vi "Test Read SD and MCP4725.vi"() -> ()   [LabVIEW 2014]
uses:
  <vilib>/LabVIEW Universal Transcriptor/MCP4725/MCP4725.lvclass
  <vilib>/LabVIEW Universal Transcriptor/LabVIEW to Arduino Transcriptor/Transcriptors/System API/Serial println string.vi
  <vilib>/LabVIEW Universal Transcriptor/LabVIEW to Arduino Transcriptor/Transcriptors/System API/Serial print integer.vi
  <vilib>/LabVIEW Universal Transcriptor/LabVIEW to Arduino Transcriptor/Transcriptors/System API/Serial print string.vi
  <vilib>/LabVIEW Universal Transcriptor/LabVIEW Universal Transcriptor SD Card Library/File.lvclass
  <vilib>/LabVIEW Universal Transcriptor/LabVIEW Universal Transcriptor SD Card Library/LabVIEW Universal Transcriptor SD Card Library.lvlib
  <vilib>/LabVIEW Universal Transcriptor/LabVIEW to Arduino Transcriptor/Transcriptors/System API/System Serial Library Variables/System Serial Library Variables.lvlib
panel:
  out "success?":bool
  out "String Buffer":string
  in  "Error In":errorcluster
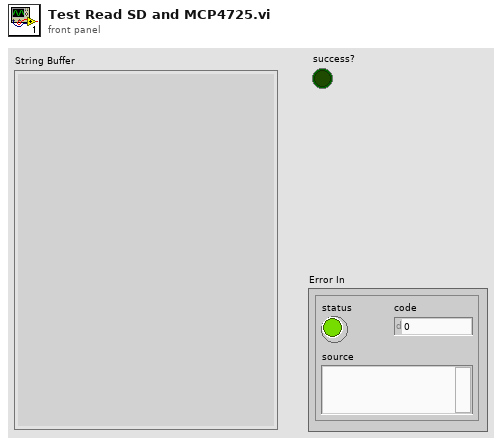
[diagram p1: front panel]
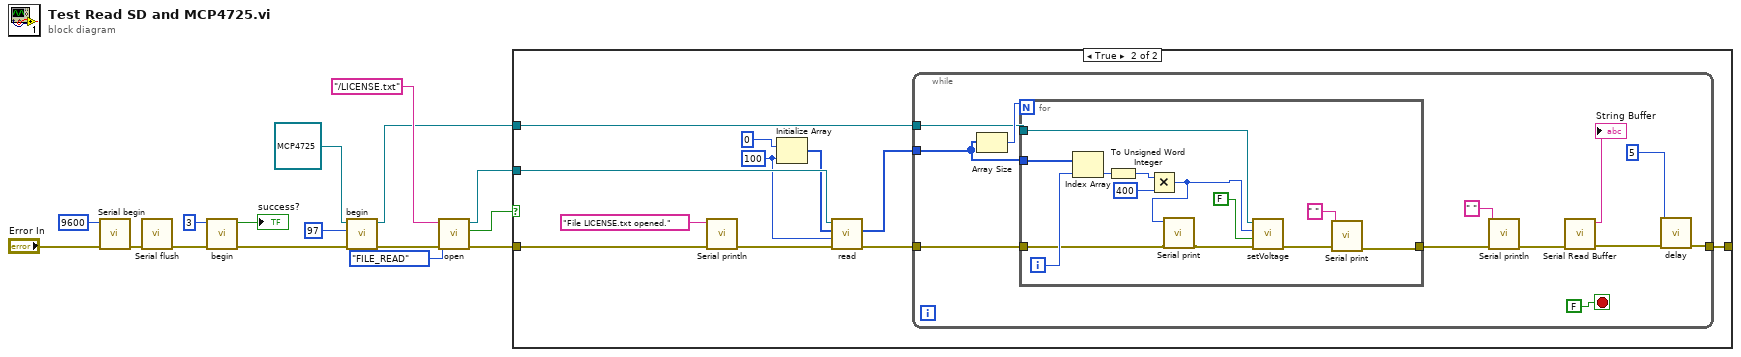
[diagram p0: block diagram]
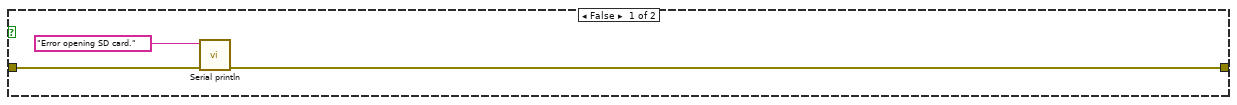
[diagram p2: hidden frame]
diagram:
  n1 = call <vilib>:"Serial begin.vi"("Error In"="Error In", "speed (Bd)"=9600) -> ("Error Out"=w4:errorcluster)  [unwired: 9 in]
  n2 = call <vilib>:"Serial flush.vi"("Error In"=w4) -> ("Error Out"=w3:errorcluster)  [unwired: 10 in]
  n3 = call <vilib>:"begin.vi"("Error In"=w3, "CS pin (optional)"=u8 3) -> ("Error Out"=w9:errorcluster, "success?"=→"success?":bool)  [unwired: 8 in]
  n4 = call <vilib>:"begin.vi"("error in (no error)"=w9, "I2C addr"=u8 97, "MCP4725 in"=refnum<class "MCP4725.lvclass"> refnum) -> ("error out"=w8:errorcluster, "MCP4725 out"=w7:refnum<class "MCP4725.lvclass">)  [unwired: 7 in]
  n5 = call <vilib>:"open.vi"("Error In"=w8, "mode"=enum16{"FILE_READ", "FILE_WRITE"}."FILE_READ", "filepath"="/LICENSE.txt") -> ("Error Out"=w11:errorcluster, "opened?"=w10:bool, "File out"=w12:refnum<class "File.lvclass">)  [unwired: 6 in]
  n6 = case shown="True" w10 {
    tunnel: w12 -> [_ w23]
    tunnel: w11 -> [w18 w30]
    tunnel: [w17 w26] -> _
    tunnel: w7 -> [_ w27]
    frame False {
      n7 = call-poly <vilib>:"Serial println.vi"("Error In"=w18, "string in"="Error opening SD card.") -> ("Error Out"=w17:errorcluster)  [unwired: 9 in]
    }
    frame True {
      w22 = 100 ("dimension size")
      n8 = call-poly <vilib>:"Serial println.vi"("Error In"=w30, "string in"="File LICENSE.txt opened.") -> ("Error Out"=w25:errorcluster)  [unwired: 9 in]
      n9 = Initialize Array(i8 0, w22) -> (w21:i8[])
      n10 = call-dynamic "read.vi"("error in (no error)"=w25, "length"=w22, "buffer"=w21, "File in"=w23) -> ("error out"=w24:errorcluster, "buffer out"=w20:i8[])  [unwired: 6 in]
      n11 = while {
        tunnel: w24 -> [w38]
        tunnel: w27 -> [w41]
        tunnel: [w33] -> w26
        tunnel: w20 -> [w37]
        stop <- FALSE stop-if-true
        n12 = Array Size(array=w37) -> (size(s)=w42:i32)
        n13 = for {
          N: w42 -> [_]
          tunnel: w38 -> [w44]
          tunnel: w37 -> [w55]
          tunnel: w41 -> [w52]
          tunnel: [w47] -> w35
          i -> [w54]
          n14 = Index Array(array=w55, index=w54) -> (element=w49:i8)
          n15 = To Unsigned Word Integer(number=w49) -> (unsigned 16bit integer=w50:u16)
          n16 = Multiply(x=w50, y=u16 400) -> (x*y=w43:u16)
          n17 = call-poly <vilib>:"Serial print.vi"("Error In"=w44, "number to print"=w43) -> ("Error Out"=w45:errorcluster)  [unwired: 9 in]
          n18 = call <vilib>:"setVoltage.vi"("error in (no error)"=w45, "writeEEPROM?"=FALSE, "voltage"=w43, "MCP4725 in"=w52) -> ("error out"=w48:errorcluster)  [unwired: 6 in, 1 out]
          n19 = call-poly <vilib>:"Serial print.vi"("Error In"=w48, "string in"=" ") -> ("Error Out"=w47:errorcluster)  [unwired: 9 in]
        }
        n20 = call-poly <vilib>:"Serial println.vi"("Error In"=w35, "string in"=" ") -> ("Error Out"=w36:errorcluster)  [unwired: 9 in]
        n21 = call <vilib>:"Serial Read Buffer.vi"("Error In"=w36) -> ("Error Out"=w32:errorcluster, "String Buffer"=→"String Buffer":string)  [unwired: 9 in]
        n22 = call <vilib>:"delay.vi"("Error In"=w32, "time (ms)"=5) -> ("Error Out"=w33:errorcluster)  [unwired: 9 in]
      }
    }
  }
